vi "Init_Instr.vi"(8 "error in (no error)":errorcluster caption="entrée d'erreur (pas d'erreur)", 11 "Class Relay_Board en entrée":refnum<class "Class Instrument UART.lvclass">) -> (0 "error out":errorcluster caption="sortie d'erreur", 3 "Class Relay_Board en Sortie":refnum<class "Class Instrument UART.lvclass">)   [LabVIEW 2020, in "Library Instrument & Equipement.lvlib" / "Library Instruments.lvlib" / "Class Instrument UART.lvclass"]
uses:
  Class Instrument UART.lvclass
  Class Instrument UART.lvclass/Class Instrument UART.ctl
  Instrument (Default)/Class Instrument (Default).lvclass
  UART/UART (Default)/Class UART (Default).lvclass
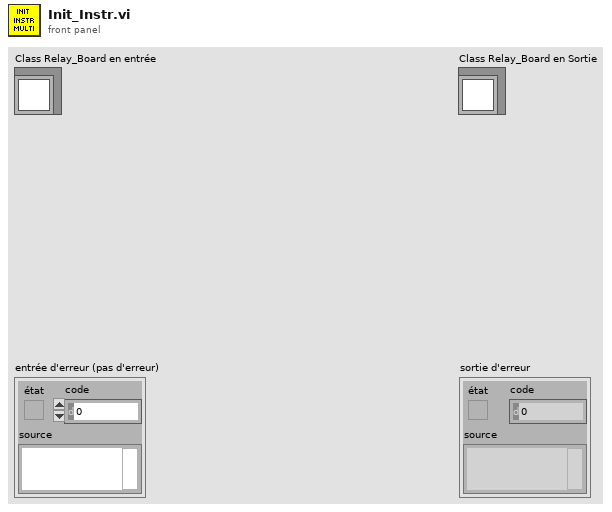
[diagram p1: front panel]
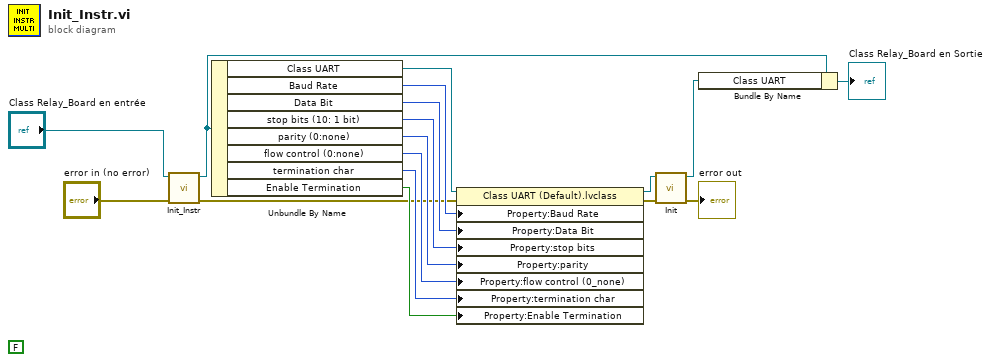
[diagram p0: block diagram]
diagram:
  (unwired) FALSE ("Autotest Ok")
  n1 = call-parent "Init_Instr.vi"("error in (no error)"="error in (no error)", "Class Instrument (Default) en entrée"="Class Relay_Board en entrée") -> ("error out"=w2:errorcluster, "Class Instrument (Default) en sortie"=w4:refnum<class "Class Instrument UART.lvclass">)  [unwired: 8 in]
  n2 = Unbundle By Name(w4) -> ("Class UART"=w12:refnum<class "Class UART (Default).lvclass">, "Baud Rate"=w11:u32, "Data Bit"=w10:u16, "stop bits (10: 1 bit)"=w9:u16, "parity (0:none)"=w8:enum16{"None", "Odd", "Even", "Mark", "Space"}, "flow control (0:none)"=w7:u16, "termination char"=w6:u8, "Enable Termination"=w5:bool)
  n3 = property class="Class UART (Default).lvclass"(reference=w12, error in=w2, "Property:Baud Rate"=w11, "Property:Data Bit"=w10, "Property:stop bits"=w9, "Property:parity"=w8, "Property:flow control (0_none)"=w7, "Property:termination char "=w6, "Property:Enable Termination"=w5) -> (reference out=w3:refnum<class "Class UART (Default).lvclass">, error out=w1:errorcluster)
  n4 = call-dynamic "Init.vi"("error in (no error)"=w1, "Class UART (Default) en entrée"=w3) -> ("error out"=→"error out":errorcluster, "Class UART (Default) en sortie"=w13:refnum<class "Class UART (Default).lvclass">)  [unwired: 8 in]
  n5 = Bundle By Name(cluster=w4, "Class UART"=w13) -> (→"Class Relay_Board en Sortie":refnum<class "Class Instrument UART.lvclass">)
